vi "max_and_min__and_select_comparator.vi"() -> ()   [LabVIEW 2019]
panel:
  out "MIN":dbl
  out "MAX.":dbl
  in  "SECOND INPUT":dbl
  in  "FIRST INPUT":dbl
  out "output":string
  in  "SWITCH":bool
  # "SELECT COMPARATOR"
  # "MAX AND MIN COMARATOR"
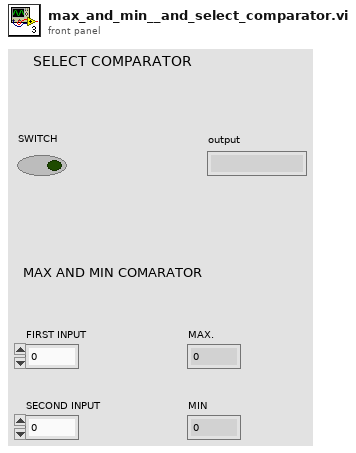
[diagram p1: front panel]
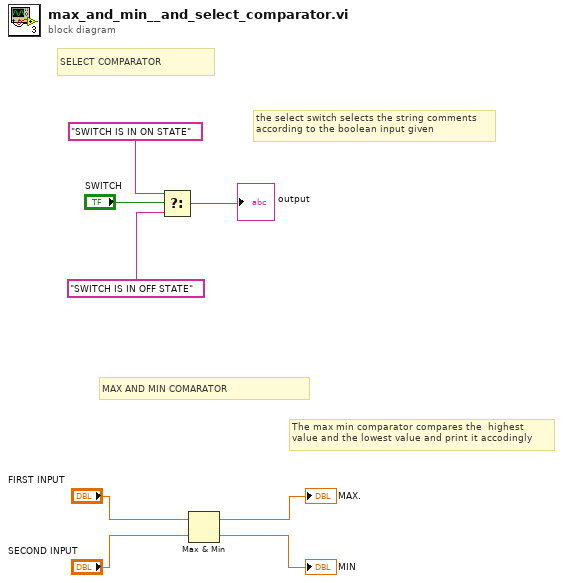
[diagram p0: block diagram]
diagram:
  # "The max min comparator compares the  highest\nvalue and the lowest value and print it accodingly"
  # "the select switch selects the string comments\naccording to the boolean input given"
  # "MAX AND MIN COMARATOR"
  # "SELECT COMPARATOR"
  n1 = Select(t="SWITCH IS IN ON STATE", s="SWITCH", f="SWITCH IS IN OFF STATE") -> (s? t:f=→"output":string)
  n2 = Max & Min(x="FIRST INPUT", y="SECOND INPUT") -> (max(x,y)=→"MAX.":dbl, min(x,y)=→"MIN":dbl)
